vi "PMC_DEMO2.vi"() -> ()   [LabVIEW 2010]
panel:
  in  "?":u16(ring) items=["+X", "-X", "+Y", "-Y"]
  in  "?":bool
  in  "Drive Speed Number":u16(ring) items=["Drive Speed 1", "Drive Speed 2", "Drive Speed 3", "Drive Speed 4"]
  out "Read Speed":u32
  in  "Set Speed":i32
  in  "?":u16(ring) items=["X", "Y"]
  in  "?":bool
  in  "?":bool
  in  "?":bool
  in  "?":bool
  in  "AXIS":u16(ring)=2 items=["X", "Y", "X,Y"]
  in  "AXIS":u16(ring)=2 items=["X", "Y", "X,Y"]
  in  "?":bool
  in  "?":u16(ring) items=["X", "Y", "X&Y"]
  in  "?":u16(ring) items=["X", "Y", "X&Y"]
  in  "?":bool
  in  "?":bool
  in  "AXIS":u16(ring) items=["X", "Y", "XY"]
  in  "Y Position(ABS)":dbl=1000.0 format="%#_8g"
  in  "X Position(ABS)":dbl=2000.0 format="%#_8g"
  in  "MOVE(ABS)":bool
  in  "MOVE(REL)":bool
  in  "X Position(REL)":dbl=1000.0 format="%#_8g"
  in  "Y Position(REL)":dbl=2000.0 format="%#_8g"
  out "MON":bool
  out "RUN (Y)":bool
  out "HOMing(Y)":bool
  out "Limit- (Y)":bool=TRUE
  out "Limit+ (Y)":bool=TRUE
  out "InPOS (Y)":bool=TRUE
  out "RUN  (X)":bool
  out "HOMing  (X)":bool
  out "Limit-  (X)":bool
  out "Limit+  (X)":bool
  out "InPOS (X)":bool=TRUE
  out "Speed(Y)":i32
  out "Speed(X)":i32
  out "Position(Y)":i32
  out "Position(X)":i32
  in  "Drive speed Set":bool
  out "Spped":u32=1000
  in  "Axis":u16(ring) items=["X", "Y"]
  in  "Drive Speed Number":u16(ring) items=["Drive Speed 1", "Drive Speed 2", "Drive Speed 3", "Drive Speed 4"]
  in  "SPEED(1~4)":string="4"
  in  "AXIS":u16(ring) items=["X", "Y"]
  in  "Speed Set":bool
  in  "BAUD(9600)":string="9600"
  in  "SET COM":bool
  out "Version":string
  in  "baud rate (9600)":u32=9600 caption="BAUD RATE(9600)"
  in  "Port":refnum<visa-resource-name>="COM4" caption="COM PORT"
  in  "SET":bool
  in  "?":bool
  # "COM SET"
  # "DRIVE SPEED SELECT"
  # "COM CHANGE"
  # "DRIVE SPEED READ"
  # "DRIVE SPEED SET"
  # "RELATIVE POSITION MOVE"
  # "MOVE STOP"
  # "CONTROLLER STATUS"
  # "ABSOLUTE POSITION MOVE"
  # "POSITION & SPEED READ"
  # "POSITION CONT CLEAR"
  # "POSITION CONT CLEAR"
  # "HOME STOP"
  # "HOME MOVE"
  # "JOG"
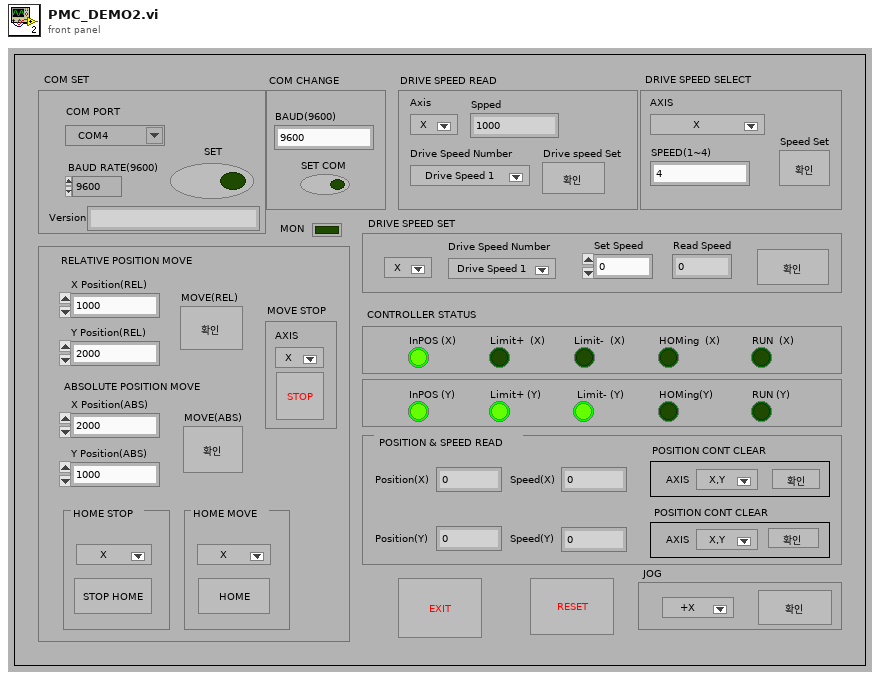
[diagram p1: front panel]
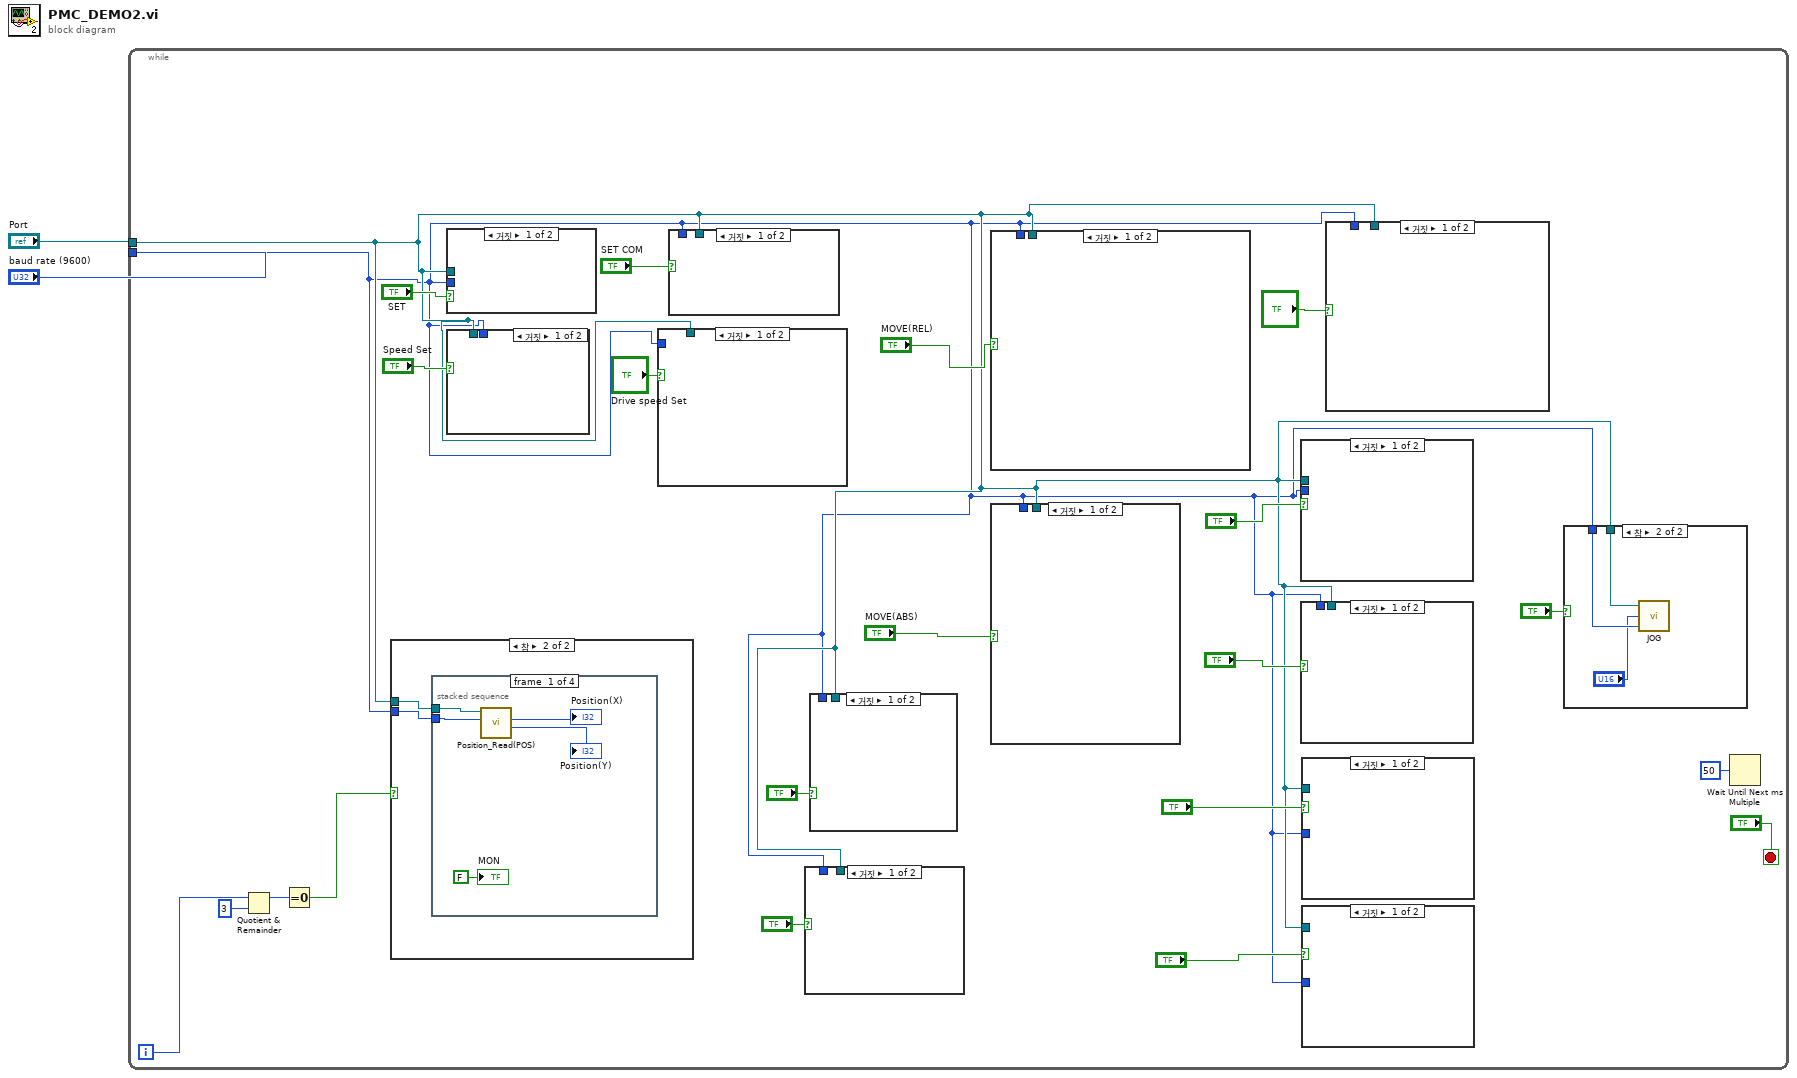
[diagram p0: block diagram]
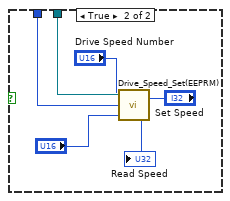
[diagram p3: hidden frame]
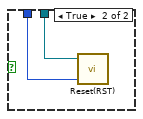
[diagram p4: hidden frame]
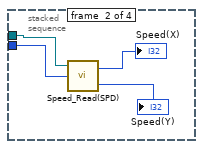
[diagram p6: hidden frame]
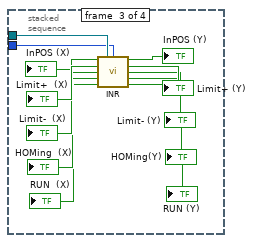
[diagram p7: hidden frame]
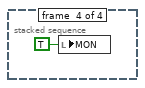
[diagram p8: hidden frame]
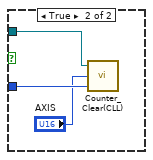
[diagram p9: hidden frame]
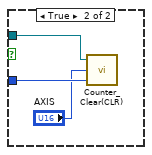
[diagram p10: hidden frame]
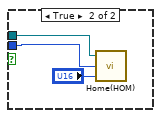
[diagram p11: hidden frame]
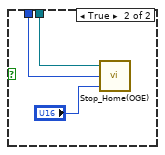
[diagram p12: hidden frame]
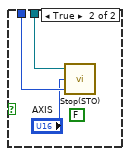
[diagram p13: hidden frame]
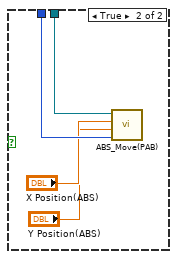
[diagram p14: hidden frame]
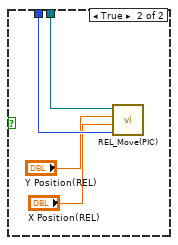
[diagram p15: hidden frame]
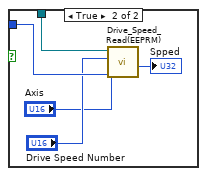
[diagram p16: hidden frame]
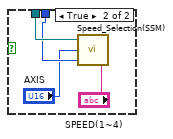
[diagram p17: hidden frame]
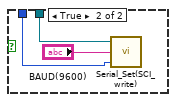
[diagram p18: hidden frame]
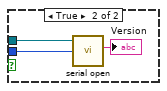
[diagram p19: hidden frame]
diagram:
  n1 = while {
    tunnel: "Port" -> [w4]
    tunnel: "baud rate (9600)" -> [w3]
    i -> [w12]
    stop <- "?" stop-if-true
    n2 = Quotient & Remainder(x=w12, y=3) -> (x-y*floor(x/y)=w10:i32)  [unwired: 1 out]
    n3 = Equal To 0?(x=w10) -> (x = 0?=w9:bool)
    n4 = case shown="참" w9 {
      tunnel: w4 -> [_ w37]
      tunnel: w3 -> [_ w36]
      frame False {
      }
      frame True {
        n5 = stacked-sequence {
          tunnel: w37 -> [w42 w46 w58 _]
          tunnel: w36 -> [w41 w45 w57 _]
          frame #0 {
            n6 = call <userlib>:"Position_Read(POS).vi"("baud rate (9600)"=w41, "Port"=w42) -> ("Position(Y)"=→"Position(Y)":i32, "Position(X)"=→"Position(X)":i32)  [unwired: 2 in, 3 out]
            "MON" <- FALSE ("MON")
          }
          frame #1 {
            n7 = call <userlib>:"Speed_Read(SPD).vi"("baud rate (9600)"=w45, "Port"=w46) -> ("Speed(Y)"=→"Speed(Y)":i32, "Speed(X)"=→"Speed(X)":i32)  [unwired: 1 in, 1 out]
          }
          frame #2 {
            n8 = call <userlib>:"INR.vi"("Port"=w58, "baud rate (9600)"=w57) -> ("InPOS (X)"=→"InPOS (X)":bool, "InPOS (Y)"=→"InPOS (Y)":bool, "Limit+  (X)"=→"Limit+  (X)":bool, "Limit+ (Y)"=→"Limit+ (Y)":bool, "Limit-  (X)"=→"Limit-  (X)":bool, "Limit- (Y)"=→"Limit- (Y)":bool, "HOMing  (X)"=→"HOMing  (X)":bool, "HOMing(Y)"=→"HOMing(Y)":bool, "RUN  (X)"=→"RUN  (X)":bool, "RUN (Y)"=→"RUN (Y)":bool)  [unwired: 4 out]
          }
          frame #3 {
            n9 = local write "MON"(TRUE ("MON")) -> ()
          }
        }
      }
    }
    n10 = case shown="거짓" "SET" {
      tunnel: w4 -> [_ w97]
      tunnel: w3 -> [_ w96]
      frame False {
      }
      frame True {
        n11 = call <userlib>:"serial open.vi"("baud rate (9600)"=w96, "Port"=w97) -> ("Version"=→"Version":string)  [unwired: 2 in, 2 out]
      }
    }
    n12 = case shown="거짓" "Speed Set" {
      tunnel: w4 -> [_ w91]
      tunnel: w3 -> [_ w90]
      frame False {
      }
      frame True {
        n13 = call <userlib>:"Speed_Selection(SSM).vi"("SPEED(1~4)"="SPEED(1~4)", "baud rate (9600)"=w90, "AXIS"="AXIS", "Port"=w91) -> ()  [unwired: 2 out]
      }
    }
    n14 = case shown="거짓" "Drive speed Set" {
      tunnel: w4 -> [_ w87]
      tunnel: w3 -> [_ w86]
      frame False {
      }
      frame True {
        n15 = call <userlib>:"Drive_Speed_Read(EEPRM).vi"("baud rate (9600)"=w86, "Axis"="Axis", "Drive Speed Number"="Drive Speed Number", "Port"=w87) -> ("Spped"=→"Spped":u32)  [unwired: 1 in, 3 out]
      }
    }
    n16 = case shown="거짓" "SET COM" {
      tunnel: w4 -> [_ w94]
      tunnel: w3 -> [_ w92]
      frame False {
      }
      frame True {
        n17 = call <userlib>:"Serial_Set(SCI_write).vi"("baud rate (9600)"=w92, "BAUD(9600)"="BAUD(9600)", "Port"=w94) -> ()  [unwired: 2 out]
      }
    }
    n18 = case shown="거짓" "?" {
      tunnel: w4 -> [_ w35]
      tunnel: w3 -> [_ w34]
      frame False {
      }
      frame True {
        n19 = call <userlib>:"Reset(RST).vi"("baud rate (9600)"=w34, "Port"=w35) -> ()  [unwired: 1 in, 2 out]
      }
    }
    n20 = case shown="거짓" "?" {
      tunnel: w4 -> [_ w74]
      tunnel: w3 -> [_ w73]
      frame False {
      }
      frame True {
        (unwired) FALSE ("mon")
        n21 = call <userlib>:"Stop(STO).vi"("baud rate (9600)"=w73, "AXIS"="AXIS", "Port"=w74) -> ()  [unwired: 2 out]
      }
    }
    n22 = case shown="거짓" "MOVE(REL)" {
      tunnel: w4 -> [_ w82]
      tunnel: w3 -> [_ w81]
      frame False {
      }
      frame True {
        n23 = call <userlib>:"REL_Move(PIC).vi"("baud rate (9600)"=w81, "X Position(REL)"="X Position(REL)", "Y Position(REL)"="Y Position(REL)", "Port"=w82) -> ()  [unwired: 1 in, 2 out]
      }
    }
    n24 = case shown="거짓" "MOVE(ABS)" {
      tunnel: w4 -> [_ w78]
      tunnel: w3 -> [_ w77]
      frame False {
      }
      frame True {
        n25 = call <userlib>:"ABS_Move(PAB).vi"("baud rate (9600)"=w77, "Y Position(ABS)"="Y Position(ABS)", "X Position(ABS)"="X Position(ABS)", "Port"=w78) -> ()  [unwired: 2 in, 3 out]
      }
    }
    n26 = case shown="거짓" "?" {
      tunnel: w4 -> [_ w68]
      tunnel: w3 -> [_ w67]
      frame False {
      }
      frame True {
        n27 = call <userlib>:"Home(HOM).vi"("AXIS"="?", "baud rate (9600)"=w67, "Port"=w68) -> ()  [unwired: 2 out]
      }
    }
    n28 = case shown="거짓" "?" {
      tunnel: w4 -> [_ w71]
      tunnel: w3 -> [_ w70]
      frame False {
      }
      frame True {
        n29 = call <userlib>:"Stop_Home(OGE).vi"("AXIS"="?", "baud rate (9600)"=w70, "Port"=w71) -> ()  [unwired: 2 out]
      }
    }
    n30 = case shown="거짓" "?" {
      tunnel: w4 -> [_ w65]
      tunnel: w3 -> [_ w64]
      frame False {
      }
      frame True {
        n31 = call <userlib>:"Counter_Clear(CLR).vi"("baud rate (9600)"=w64, "AXIS"="AXIS", "Port"=w65) -> ()  [unwired: 2 out]
      }
    }
    n32 = case shown="거짓" "?" {
      tunnel: w4 -> [_ w62]
      tunnel: w3 -> [_ w61]
      frame False {
      }
      frame True {
        n33 = call <userlib>:"Counter_Clear(CLL).vi"("baud rate (9600)"=w61, "AXIS"="AXIS", "Port"=w62) -> ()  [unwired: 2 out]
      }
    }
    n34 = case shown="거짓" "?" {
      tunnel: w4 -> [_ w33]
      tunnel: w3 -> [_ w32]
      frame False {
      }
      frame True {
        n35 = call <userlib>:"Drive_Speed_Set(EEPRM).vi"("Set Speed"="Set Speed", "Drive Speed Number"="Drive Speed Number", "Axis"="?", "baud rate (9600)"=w32, "Port"=w33) -> ("Read Speed"=→"Read Speed":u32)
      }
    }
    n36 = case shown="참" "?" {
      tunnel: w4 -> [_ w27]
      tunnel: w3 -> [_ w26]
      frame False {
      }
      frame True {
        n37 = call <userlib>:"JOG.vi"("baud rate (9600)"=w26, "AXIS"="?", "Port"=w27) -> ()  [unwired: 2 out]
      }
    }
    n38 = Wait Until Next ms Multiple(millisecond multiple=u32 50 ("ms 배수")) -> ()  [unwired: 1 out]
  }
